vi "Measurement UI.vi"() -> ()   [LabVIEW 2021, in "audio_frequencyResponseMeasurement.lvlib"]
uses:
  audio_frequencyResponseMeasurement.lvlib
panel:
  in  "MeasGraphs":T1(tab)
  out "FrequencyResponseGraph":cluster{"X":dbl[], "Y":dbl[]}(graph) caption="AC"
  out "TimeDomainGraph":waveform(dbl)(graph) caption="AC"
  out "RMSLevelGraph":cluster{"X":dbl[], "Y":dbl[]}(graph) caption="AC"
  out "THDResponseGraph":cluster{"X":dbl[], "Y":dbl[]}(graph) caption="AC"
  out "THD+NResponseGraph":cluster{"X":dbl[], "Y":dbl[]}(graph) caption="AC"
  out "THD+N response":dbl[](array[numeric])
  out "Frequency response":dbl[](array[numeric])
  out "Time domain":dbl[](array[numeric])
  out "dt":dbl
  in  "Analog source resource name":string
  in  "Protocol capture channel":string="0L" caption="Channel list"
  out "RMS levels":dbl[](array[numeric])
  out "Harmonics levels":dbl[](array[numeric])
  out "THD response":dbl[](array[numeric])
  out "Frequency steps":dbl[](array[numeric])
  in  "Data line":u16 caption="DATA LINE"
  in  "Channel":u32 caption="CHANNEL"
  in  "MeasSettingsOptions":i32(listbox)=-1
  in  "Settling time":dbl caption="SETTLING TIME" format="%#_6ps"
  in  "Setting cycles":i32 caption="SETTLING CYCLES"
  in  "Maximum harmonic":i32=5 caption="MAX HARMONIC"
  in  "DC Offset":dbl caption="DC OFFSET" format="%#_6pV"
  out "Calculated sample rate":u32 caption="SAMPLE RATE" format="%#.6pHz"
  in  "Trigger source":T2(ring) caption="TRIGGER SOURCE"
  in  "Protocol capture resource name":string caption="RESOURCE NAME"
  out "Protocol settings":string="Protocol settings"
  in  "Clock rate":u32=2822400 caption="CLOCK RATE" format="%#.6pHz"
  in  "Frequency spacing":enum16{"Linear", "Logarithmic"}(ring)=enum."Logarithmic" caption="FREQUENCY SPACING"
  in  "Measurement duration":dbl=0.001 caption="MEASUREMENT DURATION" format="%#_6ps"
  in  "Measurement cycles":i32=10 caption="MEASUREMENT CYCLES"
  in  "Frequency steps":i32=20 caption="FREQUENCY STEPS"
  out "Analog source":string="Analog source "
  in  "DSGResourceName":tag="<Select Device>" caption="RESOURCE NAME"
  in  "Amplitude":dbl=-1.0 caption="AMPLITUDE" format="%#_6pdB"
  in  "Full scale range":dbl=3.16 caption="FULL SCALE RANGE" format="%.3pV"
  in  "Frequency stop":dbl=10000.0 caption="FREQUENCY STOP" format="%#_6pHz"
  in  "Frequency start":dbl=100.0 caption="FREQUENCY START" format="%#_6pHz"
  out "Measurement settings":string="Measurement settings"
  in  "MeasSettings":bool
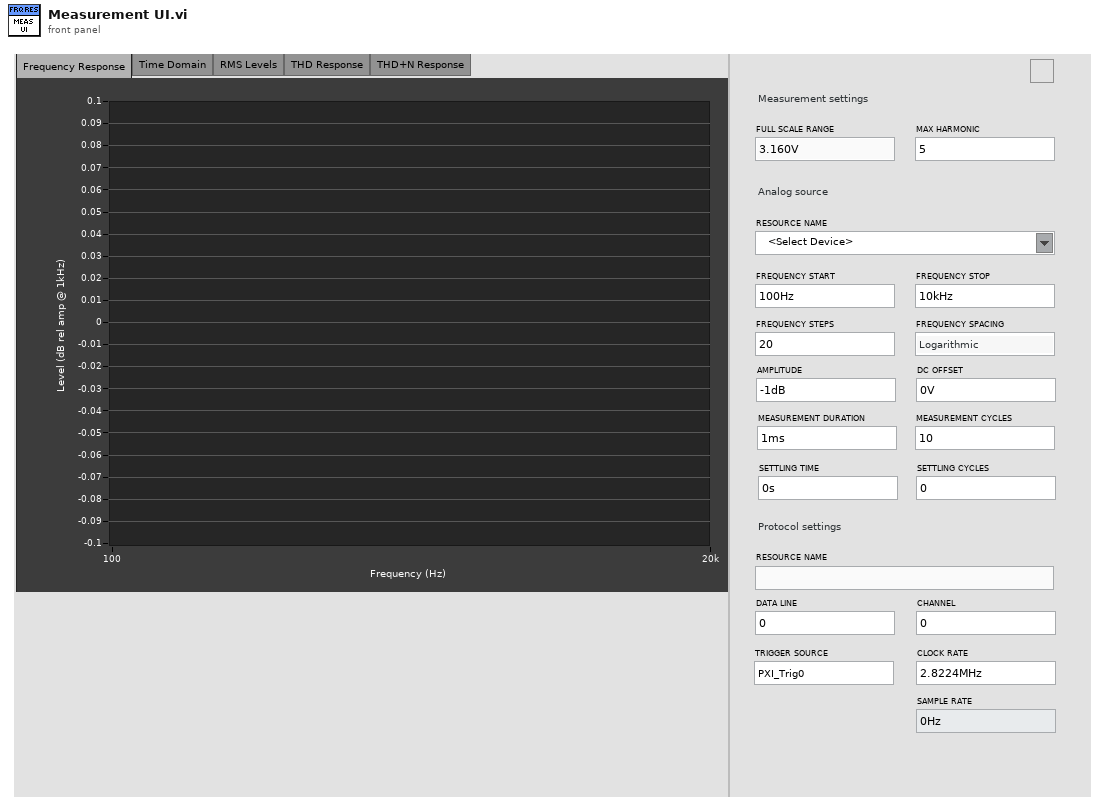
[diagram p1: front panel]
types:
  T1 = enum32{"Frequency Response", "Time Domain", "RMS Levels", "THD Response", "THD+N Response", "Hidden Controls"}
  T2 = enum16{"PXI_Trig0", "PXI_Trig1", "PXI_Trig2", "PXI_Trig3", "PXI_Trig4", "PXI_Trig5", "PXI_Trig6", "PXI_Trig7"}
  T3 = enum16{"open", "replace", "create", "open or create", "replace or create", "replace or create with confirmation"}
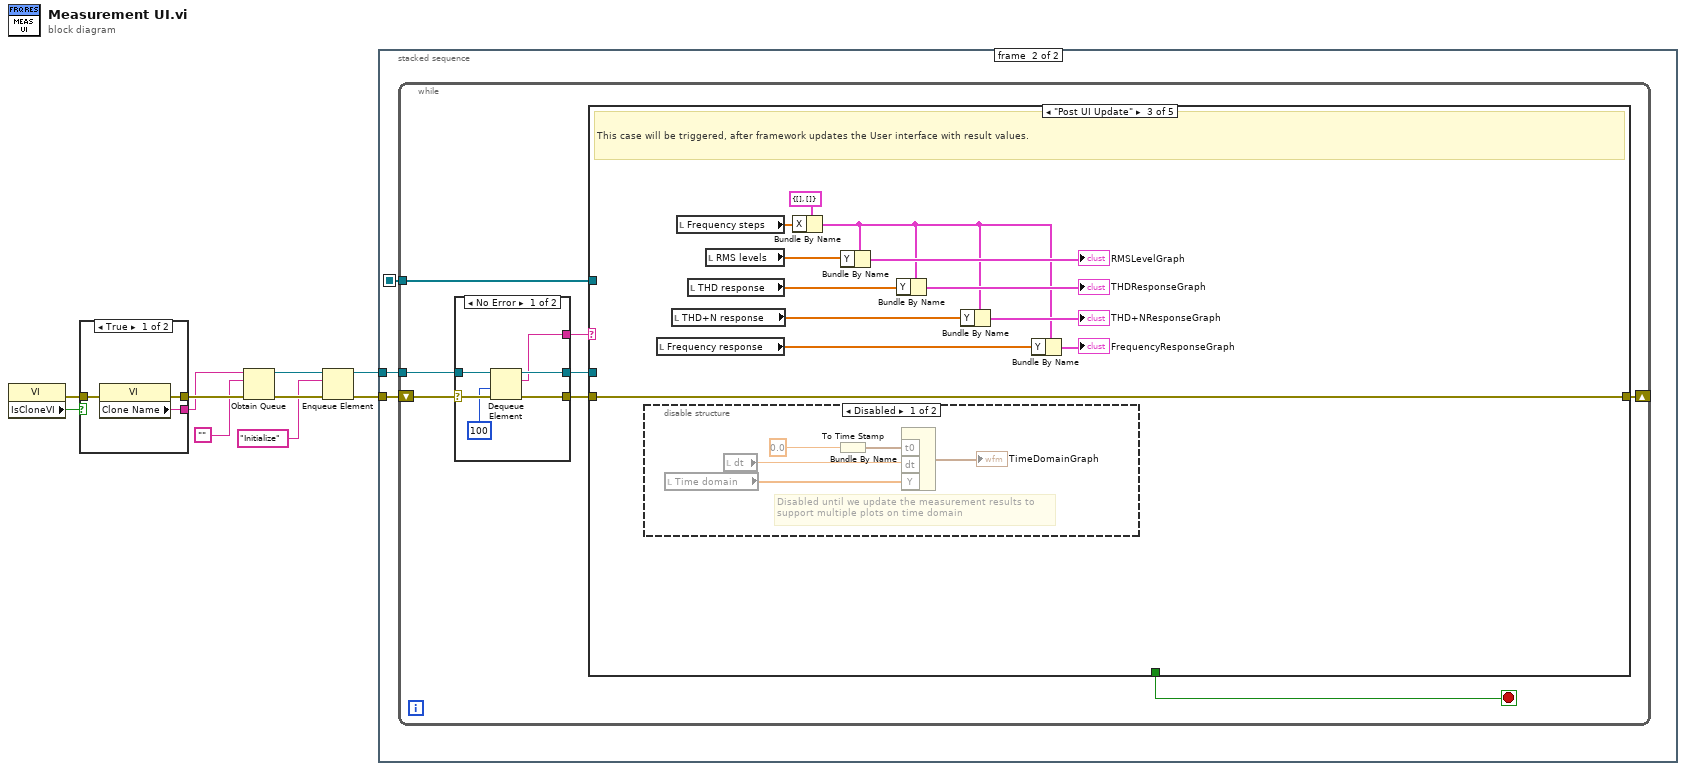
[diagram p0: block diagram]
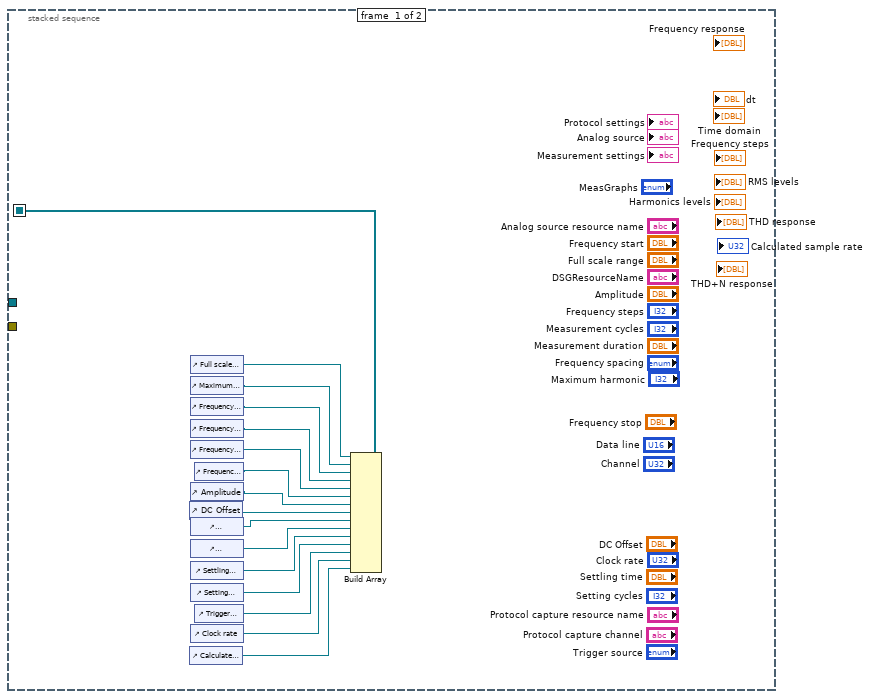
[diagram p2: hidden frame]
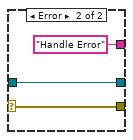
[diagram p3: hidden frame]
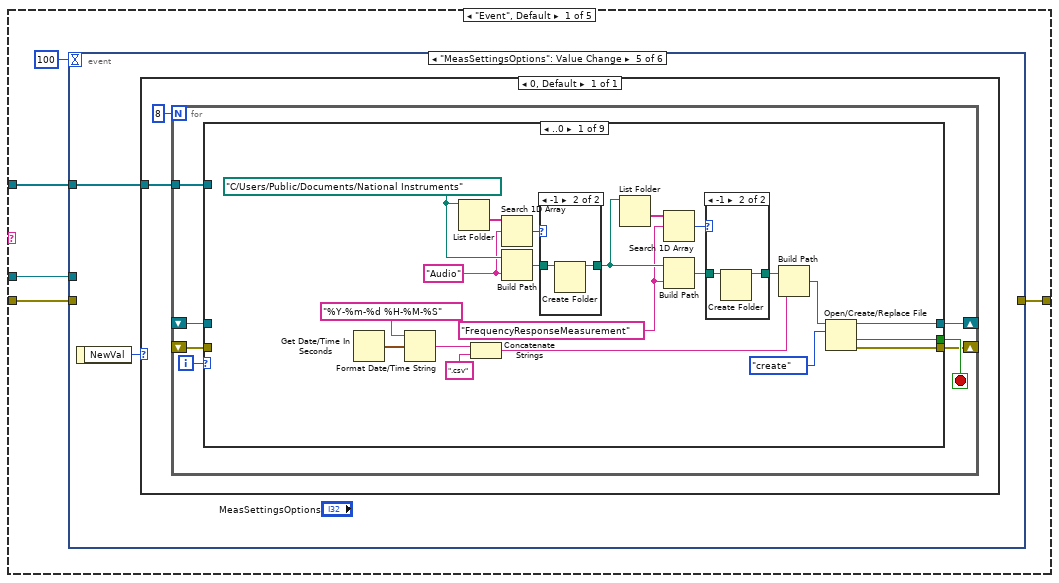
[diagram p4: hidden frame]
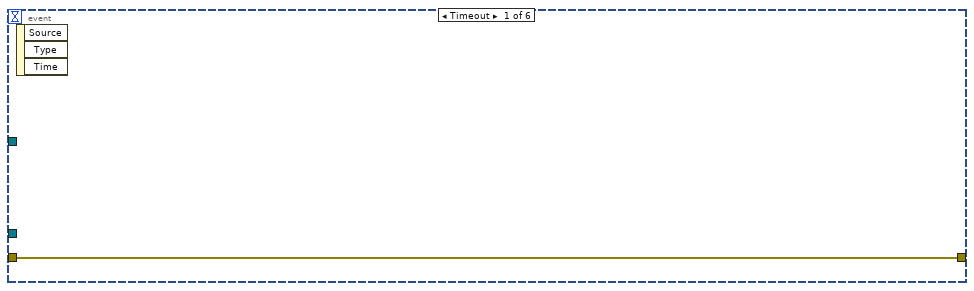
[diagram p5: hidden frame]
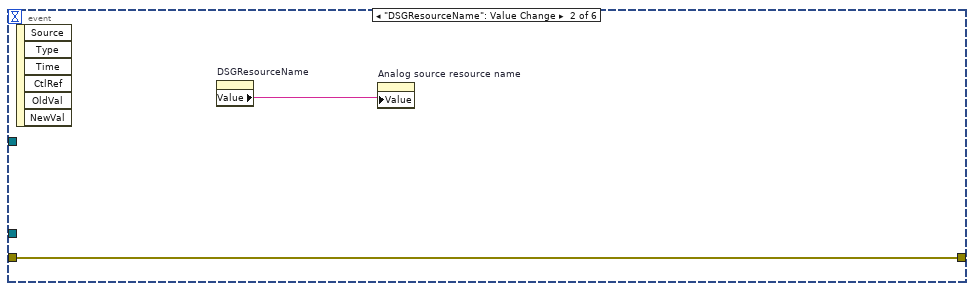
[diagram p6: hidden frame]
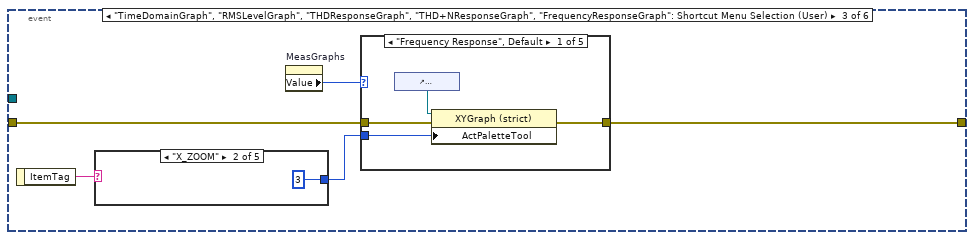
[diagram p7: hidden frame]
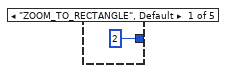
[diagram p8: hidden frame]
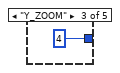
[diagram p9: hidden frame]
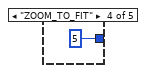
[diagram p10: hidden frame]
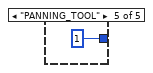
[diagram p11: hidden frame]
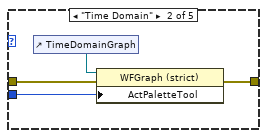
[diagram p12: hidden frame]
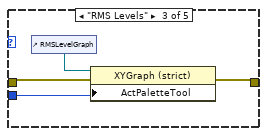
[diagram p13: hidden frame]
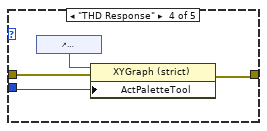
[diagram p14: hidden frame]
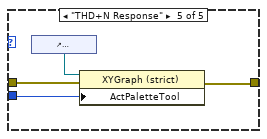
[diagram p15: hidden frame]
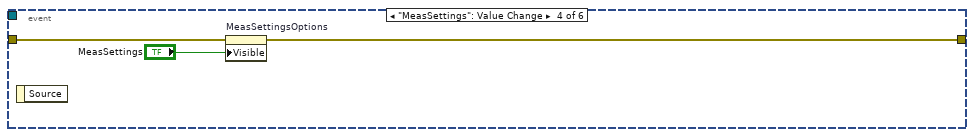
[diagram p16: hidden frame]
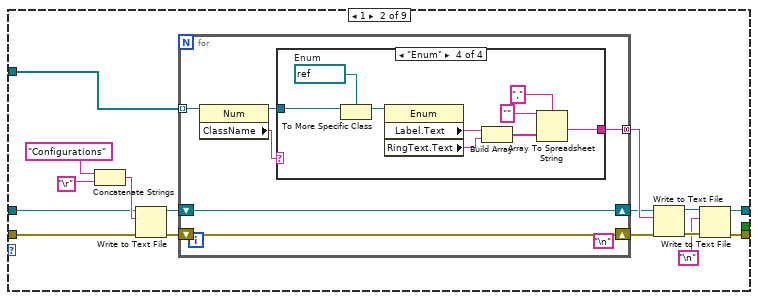
[diagram p19: hidden frame]
diagram:
  n1 = property class="VI"() -> (error out=w1:errorcluster, "IsCloneVI"=w2:bool)  [unwired: 2 in, 1 out]
  n2 = case shown="True" w2 {
    tunnel: [w13 w16] -> w10
    tunnel: [w12 w15] -> w9
    tunnel: w1 -> [w11 w14]
    frame True {
      n3 = property class="VI"(error in=w11) -> (error out=w13:errorcluster, "Clone Name"=w12:string)  [unwired: 1 in, 1 out]
    }
    frame False {
      n4 = property class="VI"(error in=w14) -> (error out=w16:errorcluster, "Name"=w15:string)  [unwired: 1 in, 1 out]
    }
  }
  n5 = Obtain Queue(name (unnamed)=w9, element data type="", error in (no error)=w10) -> (queue out=w6:refnum<queue>, error out=w8:errorcluster)  [unwired: 2 in, 1 out]
  n6 = Enqueue Element(queue=w6, element="Initialize", error in (no error)=w8) -> (queue out=w5:refnum<queue>, error out=w7:errorcluster)  [unwired: 1 in, 1 out]
  n7 = stacked-sequence {
    seq-local: [w19 _] -> [_ w33]
    tunnel: w7 -> [_ w35]
    tunnel: w5 -> [_ w34]
    frame #0 {
      n8 = control-ref of="DC Offset"() -> (w17:refnum<vi>)
      n9 = control-ref of="Calculated sample rate"() -> (w20:refnum<vi>)
      n10 = control-ref of="Full scale range"() -> (w32:refnum<vi>)
      n11 = control-ref of="Maximum harmonic"() -> (w31:refnum<vi>)
      n12 = control-ref of="Frequency start"() -> (w30:refnum<vi>)
      n13 = control-ref of="Frequency stop"() -> (w29:refnum<vi>)
      n14 = control-ref of="Frequency steps"() -> (w28:refnum<vi>)
      n15 = control-ref of="Amplitude"() -> (w18:refnum<vi>)
      n16 = control-ref of="Measurement duration"() -> (w26:refnum<vi>)
      n17 = control-ref of="Measurement cycles"() -> (w25:refnum<vi>)
      n18 = control-ref of="Settling time"() -> (w24:refnum<vi>)
      n19 = control-ref of="Setting cycles"() -> (w23:refnum<vi>)
      n20 = control-ref of="Clock rate"() -> (w21:refnum<vi>)
      n21 = control-ref of="Frequency spacing"() -> (w27:refnum<vi>)
      n22 = control-ref of="Trigger source"() -> (w22:refnum<vi>)
      n23 = Build Array(w32, w31, w30, w29, w28, w27, w18, w17, w26, w25, w24, w23, w22, w21, w20) -> (w19:refnum<vi>[])
    }
    frame #1 {
      n24 = while {
        shift-right: [w38] -> _
        shift-left: w35 -> [w43]
        tunnel: w34 -> [w41]
        tunnel: w33 -> [w36]
        stop <- w37 stop-if-true
        n25 = case shown="No Error" w43 {
          selector: w43 -> [w49 w52]
          tunnel: [w48 w52] -> w42
          tunnel: w41 -> [w47 w51]
          tunnel: [w46 w51] -> w40
          tunnel: [w45 "Handle Error"] -> w39
          frame No Error {
            n26 = Dequeue Element(queue=w47, timeout in ms (-1)=100, error in (no error)=w49) -> (queue out=w46:refnum<queue>, element=w45:string, error out=w48:errorcluster)  [unwired: 1 out]
          }
          frame Error {
          }
        }
        n27 = case shown="\"Post UI Update\"" w39 {
          tunnel: w42 -> [w56 w365 w379 w391 w392]
          tunnel: w40 -> [w54 _ _ w389 _]
          tunnel: [w57 w365 w379 w386 w392] -> w38
          tunnel: [_ _ _ TRUE _] -> w37
          tunnel: w36 -> [w53 _ _ _ _]
          frame "Event", Default {
            n28 = event shown="[4] \"MeasSettingsOptions\": Value Change" {
              selector: _ -> [_ _ _ _ _ _]
              dyn-events: _ -> [_ _ _ _ _ _]
              timeout: 100 -> [_ _ _ _ _ _]
              tunnel: [w58 w60 w61 w91 _ w354] -> w57
              tunnel: w56 -> [w58 w60 w63 w93 _ w355]
              tunnel: w54 -> [_ _ _ _ _ w353]
              tunnel: w53 -> [_ _ _ _ w95 _]
              event Timeout {
                n29 = event-data() -> ()  [unwired: 1 in, 3 out]
              }
              event "DSGResourceName": Value Change {
                n30 = event-data() -> ()  [unwired: 1 in, 6 out]
                n31 = property on="DSGResourceName" class="DAQmxName"() -> ("Value"=w59:string)  [unwired: 2 in, 2 out]
                n32 = property on="Analog source resource name" class="Str"("Value"=w59) -> ()  [unwired: 2 in, 2 out]
              }
              event "TimeDomainGraph", "RMSLevelGraph", "THDResponseGraph", "THD+NResponseGraph", "FrequencyResponseGraph": Shortcut Menu Selection (User) {
                n33 = event-data() -> ("ItemTag"=w64:string)  [unwired: 1 in]
                n34 = case shown="\"X_ZOOM\"" w64 {
                  tunnel: [2 3 4 5 1] -> w62
                  frame "ZOOM_TO_RECTANGLE", Default {
                  }
                  frame "X_ZOOM" {
                  }
                  frame "Y_ZOOM" {
                  }
                  frame "ZOOM_TO_FIT" {
                  }
                  frame "PANNING_TOOL" {
                  }
                }
                n35 = property on="MeasGraphs" class="TabCtl (strict)"() -> ("Value"=w65:T1)  [unwired: 2 in, 2 out]
                n36 = case shown="\"Frequency Response\", Default" w65 {
                  tunnel: w63 -> [w74 w77 w81 w86 w90]
                  tunnel: w62 -> [w71 w76 w80 w83 w89]
                  tunnel: [w73 w75 w79 w85 w88] -> w61
                  frame "Frequency Response", Default {
                    n37 = control-ref of="FrequencyResponseGraph"() -> (w72:refnum<vi>)
                    n38 = property class="XYGraph (strict)"(reference=w72, error in=w74, "ActPaletteTool"=w71) -> (error out=w73:errorcluster)  [unwired: 1 out]
                  }
                  frame "Time Domain" {
                    n39 = control-ref of="TimeDomainGraph"() -> (w78:refnum<vi>)
                    n40 = property class="WFGraph (strict)"(reference=w78, error in=w77, "ActPaletteTool"=w76) -> (error out=w75:errorcluster)  [unwired: 1 out]
                  }
                  frame "RMS Levels" {
                    n41 = control-ref of="RMSLevelGraph"() -> (w82:refnum<vi>)
                    n42 = property class="XYGraph (strict)"(reference=w82, error in=w81, "ActPaletteTool"=w80) -> (error out=w79:errorcluster)  [unwired: 1 out]
                  }
                  frame "THD Response" {
                    n43 = control-ref of="THDResponseGraph"() -> (w84:refnum<vi>)
                    n44 = property class="XYGraph (strict)"(reference=w84, error in=w86, "ActPaletteTool"=w83) -> (error out=w85:errorcluster)  [unwired: 1 out]
                  }
                  frame "THD+N Response" {
                    n45 = control-ref of="THD+NResponseGraph"() -> (w87:refnum<vi>)
                    n46 = property class="XYGraph (strict)"(reference=w87, error in=w90, "ActPaletteTool"=w89) -> (error out=w88:errorcluster)  [unwired: 1 out]
                  }
                }
              }
              event "MeasSettings": Value Change {
                n47 = event-data() -> ()  [unwired: 1 in, 1 out]
                n48 = property on="MeasSettingsOptions" class="LstBox (strict)"(error in=w93, "Visible"="MeasSettings") -> (error out=w91:errorcluster)  [unwired: 1 in, 1 out]
              }
              event "MeasSettingsOptions": Value Change {
                n49 = event-data() -> ("NewVal"=w94:i32)  [unwired: 1 in]
                n50 = case shown="0, Default" w94 {
                  tunnel: w95 -> [w96]
                  frame 0, Default {
                    n51 = for {
                      N: 8 -> [_]
                      shift-right: [w102] -> _
                      shift-left: _ -> [w101]
                      shift-right: [w100] -> _
                      shift-left: _ -> [w99]
                      tunnel: w96 -> [w98]
                      i -> [w104]
                      stop <- w103 stop-if-true
                      n52 = case shown="..0" w104 {
                        tunnel: [w118 _ _ _ _ _ _ _ _] -> w103
                        tunnel: [w124 w144 w188 w215 w253 w285 w317 refnum<file> refnum ("refnum out") w351] -> w102
                        tunnel: w101 -> [_ w141 w208 w226 w274 w306 w338 w349 w351]
                        tunnel: [w117 w143 w186 w214 w251 w283 w315 w347 w350] -> w100
                        tunnel: w99 -> [_ w139 w207 w227 w273 w305 w337 w346 w350]
                        tunnel: w98 -> [_ w142 _ _ _ _ _ _ _]
                        frame ..0 {
                          w113 = "FrequencyResponseMeasurement" ("prompt")
                          w120 = "Audio" ("prompt")
                          w123 = path "C:/Users/Public/Documents/National Instruments" ("base path")
                          n53 = Get Date/Time In Seconds() -> (seconds since 1Jan1904=w110:timestamp)
                          n54 = Format Date/Time String(time format string (%c)="%Y-%m-%d %H-%M-%S", seconds (now)=w110) -> (date/time string=w109:string)  [unwired: 1 in]
                          n55 = List Folder(path=w123) -> (folder names=w121:string[])  [unwired: 3 in, 3 out]
                          n56 = Concatenate Strings(w109, ".csv" ("string")) -> (w106:string)
                          n57 = Search 1D Array(1D array=w121, element=w120) -> (index of element=w119:i32)  [unwired: 1 in]
                          n58 = Build Path(base path=w123, name or relative path=w120) -> (appended path=w122:path)
                          n59 = case shown="-1" w119 {
                            tunnel: w122 -> [w129 w131]
                            tunnel: [w129 w130] -> w114
                            frame Default {
                            }
                            frame -1 {
                              n60 = Create Folder(path (use dialog)=w131) -> (created path=w130:path)  [unwired: 2 in, 2 out]
                            }
                          }
                          n61 = List Folder(path=w114) -> (folder names=w116:string[])  [unwired: 3 in, 3 out]
                          n62 = Search 1D Array(1D array=w116, element=w113) -> (index of element=w115:i32)  [unwired: 1 in]
                          n63 = Build Path(base path=w114, name or relative path=w113) -> (appended path=w112:path)
                          n64 = case shown="-1" w115 {
                            tunnel: w112 -> [w126 w128]
                            tunnel: [w126 w127] -> w107
                            frame Default {
                            }
                            frame -1 {
                              n65 = Create Folder(path (use dialog)=w128) -> (created path=w127:path)  [unwired: 2 in, 2 out]
                            }
                          }
                          n66 = Build Path(base path=w107, name or relative path=w106) -> (appended path=w105:path)
                          n67 = Open/Create/Replace File(file path (use dialog)=w105, operation (0:open)=T3."create") -> (refnum out=w124:refnum<file>, cancelled=w118:bool, error out=w117:errorcluster)  [unwired: 4 in]
                        }
                        frame 1 {
                          (unwired) "\n"
                          n68 = Concatenate Strings("Configurations" ("format string"), "\r") -> (w145:string)
                          n69 = Write to Text File(file (use dialog)=w141, text=w145, error in=w139) -> (refnum out=w138:refnum<file>, error out=w140:errorcluster)  [unwired: 1 in, 1 out]
                          n70 = for {
                            tunnel: w142 -> [w149] mode=indexing
                            shift-right: [w153] -> w136
                            shift-left: w138 -> [w153]
                            shift-right: [w152] -> w135
                            shift-left: w140 -> [w152]
                            tunnel: [w151] -> w137 mode=concatenating
                            n71 = property class="Num"(reference=w149) -> (reference out=w150:refnum<vi>, "ClassName"=w148:string)  [unwired: 1 in, 1 out]
                            n72 = case shown="\"Enum\"" w148 {
                              tunnel: [_ w157 w167 w176] -> w151
                              tunnel: w150 -> [_ w155 w165 w180]
                              frame Default {
                              }
                              frame "Digital" {
                                w154 = refnum<vi> refnum  # Digital
                                n73 = To More Specific Class(target class=w154, reference=w155) -> (specific class reference=w156:refnum<vi>)  [unwired: 1 in, 1 out]
                                n74 = property class="DigNum"(reference=w156) -> ("Label.Text"=w162:string, "NumText.Text"=w161:string)  [unwired: 1 in, 2 out]
                                n75 = Build Array(w162, w161) -> (w158:string[])
                                n76 = Array To Spreadsheet String(delimiter (Tab)=",", array=w158, 3:"" ("format string")) -> (spreadsheet string=w157:string)
                              }
                              frame "Ring" {
                                w164 = refnum<vi> refnum  # Ring
                                n77 = To More Specific Class(target class=w164, reference=w165) -> (specific class reference=w166:refnum<vi>)  [unwired: 1 in, 1 out]
                                n78 = property class="Ring"(reference=w166) -> ("Label.Text"=w163:string, "RingText.Text"=w171:string)  [unwired: 1 in, 2 out]
                                n79 = Build Array(w163, w171) -> (w168:string[])
                                n80 = Array To Spreadsheet String(delimiter (Tab)=",", array=w168, 3:"" ("format string")) -> (spreadsheet string=w167:string)
                              }
                              frame "Enum" {
                                w179 = refnum<vi> refnum  # Enum
                                n81 = To More Specific Class(target class=w179, reference=w180) -> (specific class reference=w175:refnum<vi>)  [unwired: 1 in, 1 out]
                                n82 = property class="Enum"(reference=w175) -> ("Label.Text"=w174:string, "RingText.Text"=w173:string)  [unwired: 1 in, 2 out]
                                n83 = Build Array(w174, w173) -> (w172:string[])
                                n84 = Array To Spreadsheet String(delimiter (Tab)=",", array=w172, 3:"" ("format string")) -> (spreadsheet string=w176:string)
                              }
                            }
                          }
                          n85 = Write to Text File(file (use dialog)=w136, text=w137, error in=w135) -> (refnum out=w134:refnum<file>, error out=w133:errorcluster)  [unwired: 1 in, 1 out]
                          n86 = Write to Text File(file (use dialog)=w134, text="\n", error in=w133) -> (refnum out=w144:refnum<file>, error out=w143:errorcluster)  [unwired: 1 in, 1 out]
                        }
                        frame 2 {
                          w181 = "\r"
                          n87 = property on="FrequencyResponseGraph" class="XYGraph (strict)"() -> ("Value"=w183:cluster{"X":dbl[], "Y":dbl[]})  [unwired: 2 in, 2 out]
                          n88 = Concatenate Strings("Results" ("string"), w181, "Frequency Response" ("string"), w181) -> (w205:string)
                          n89 = Write to Text File(file (use dialog)=w208, text=w205, error in=w207) -> (refnum out=w201:refnum<file>, error out=w200:errorcluster)  [unwired: 1 in, 1 out]
                          n90 = Build Array("Frequency (Hz)", "Level (dB rel amp @ 1kHz)") -> (w204:string[])
                          n91 = Unbundle By Name(w183) -> ("X"=w192:dbl[], "Y"=w193:dbl[])
                          n92 = Array To Spreadsheet String(delimiter (Tab)=",", array=w204, 3:"" ("format string")) -> (spreadsheet string=w199:string)
                          n93 = for {
                            tunnel: w192 -> [w213] mode=indexing
                            tunnel: w193 -> [w209] mode=indexing
                            tunnel: [w210] -> w194 mode=indexing
                            n94 = Format Into String(w213) -> (resulting string=w211:string)  [unwired: 3 in, 1 out]
                            n95 = Format Into String(w209) -> (resulting string=w212:string)  [unwired: 3 in, 1 out]
                            n96 = Build Array(w211, w212) -> (w210:string[])
                          }
                          n97 = Write to Text File(file (use dialog)=w201, text=w199, error in=w200) -> (refnum out=w198:refnum<file>, error out=w197:errorcluster)  [unwired: 1 in, 1 out]
                          n98 = Array To Spreadsheet String(delimiter (Tab)=",", array=w194, 3:"" ("format string")) -> (spreadsheet string=w191:string)
                          n99 = Write to Text File(file (use dialog)=w198, text=w191, error in=w197) -> (refnum out=w190:refnum<file>, error out=w189:errorcluster)  [unwired: 1 in, 1 out]
                          n100 = Write to Text File(file (use dialog)=w190, text="\n", error in=w189) -> (refnum out=w188:refnum<file>, error out=w186:errorcluster)  [unwired: 1 in, 1 out]
                        }
                        frame 3 {
                          n101 = property on="TimeDomainGraph" class="WFGraph (strict)"() -> ("Value"=w219:waveform(dbl))  [unwired: 2 in, 2 out]
                          n102 = Concatenate Strings("Time Domain" ("string"), "\r") -> (w239:string)
                          n103 = Write to Text File(file (use dialog)=w226, text=w239, error in=w227) -> (refnum out=w236:refnum<file>, error out=w235:errorcluster)  [unwired: 1 in, 1 out]
                          n104 = Build Array("Time (s)", "Amplitude (V)") -> (w238:string[])
                          n105 = Unbundle By Name(w219) -> ("dt"=w224:dbl, "Y"=w225:dbl[])
                          n106 = Array To Spreadsheet String(delimiter (Tab)=",", array=w238, 3:"" ("format string")) -> (spreadsheet string=w234:string)
                          n107 = Write to Text File(file (use dialog)=w236, text=w234, error in=w235) -> (refnum out=w233:refnum<file>, error out=w232:errorcluster)  [unwired: 1 in, 1 out]
                          n108 = for {
                            tunnel: [w245] -> w229 mode=indexing
                            tunnel: w225 -> [w244] mode=indexing
                            tunnel: w224 -> [w242]
                            i -> [w243]
                            n109 = Multiply(x=w242, y=w243) -> (x*y=w241:dbl)
                            n110 = Format Into String(w241) -> (resulting string=w246:string)  [unwired: 3 in, 1 out]
                            n111 = Format Into String(w244) -> (resulting string=w247:string)  [unwired: 3 in, 1 out]
                            n112 = Build Array(w246, w247) -> (w245:string[])
                          }
                          n113 = Array To Spreadsheet String(delimiter (Tab)=",", array=w229, 3:"" ("format string")) -> (spreadsheet string=w228:string)
                          n114 = Write to Text File(file (use dialog)=w233, text=w228, error in=w232) -> (refnum out=w217:refnum<file>, error out=w216:errorcluster)  [unwired: 1 in, 1 out]
                          n115 = Write to Text File(file (use dialog)=w217, text="\n", error in=w216) -> (refnum out=w215:refnum<file>, error out=w214:errorcluster)  [unwired: 1 in, 1 out]
                        }
                        frame 4 {
                          n116 = property on="RMSLevelGraph" class="XYGraph (strict)"() -> ("Value"=w248:cluster{"X":dbl[], "Y":dbl[]})  [unwired: 2 in, 2 out]
                          n117 = Concatenate Strings("RMS Level" ("string"), "\r") -> (w271:string)
                          n118 = Build Array("Frequency (Hz)", "Level (Vrms)") -> (w270:string[])
                          n119 = Write to Text File(file (use dialog)=w274, text=w271, error in=w273) -> (refnum out=w267:refnum<file>, error out=w266:errorcluster)  [unwired: 1 in, 1 out]
                          n120 = Array To Spreadsheet String(delimiter (Tab)=",", array=w270, 3:"" ("format string")) -> (spreadsheet string=w265:string)
                          n121 = Unbundle By Name(w248) -> ("X"=w258:dbl[], "Y"=w259:dbl[])
                          n122 = Write to Text File(file (use dialog)=w267, text=w265, error in=w266) -> (refnum out=w264:refnum<file>, error out=w263:errorcluster)  [unwired: 1 in, 1 out]
                          n123 = for {
                            tunnel: w258 -> [w279] mode=indexing
                            tunnel: w259 -> [w275] mode=indexing
                            tunnel: [w276] -> w260 mode=indexing
                            n124 = Format Into String(w279) -> (resulting string=w277:string)  [unwired: 3 in, 1 out]
                            n125 = Format Into String(w275) -> (resulting string=w278:string)  [unwired: 3 in, 1 out]
                            n126 = Build Array(w277, w278) -> (w276:string[])
                          }
                          n127 = Array To Spreadsheet String(delimiter (Tab)=",", array=w260, 3:"" ("format string")) -> (spreadsheet string=w257:string)
                          n128 = Write to Text File(file (use dialog)=w264, text=w257, error in=w263) -> (refnum out=w255:refnum<file>, error out=w254:errorcluster)  [unwired: 1 in, 1 out]
                          n129 = Write to Text File(file (use dialog)=w255, text="\n", error in=w254) -> (refnum out=w253:refnum<file>, error out=w251:errorcluster)  [unwired: 1 in, 1 out]
                        }
                        frame 5 {
                          n130 = Concatenate Strings("THD Response" ("string"), "\r") -> (w303:string)
                          n131 = property on="THDResponseGraph" class="XYGraph (strict)"() -> ("Value"=w280:cluster{"X":dbl[], "Y":dbl[]})  [unwired: 2 in, 2 out]
                          n132 = Build Array("Frequency (Hz)", "THD (dB)") -> (w302:string[])
                          n133 = Write to Text File(file (use dialog)=w306, text=w303, error in=w305) -> (refnum out=w299:refnum<file>, error out=w298:errorcluster)  [unwired: 1 in, 1 out]
                          n134 = Array To Spreadsheet String(delimiter (Tab)=",", array=w302, 3:"" ("format string")) -> (spreadsheet string=w297:string)
                          n135 = Unbundle By Name(w280) -> ("X"=w290:dbl[], "Y"=w291:dbl[])
                          n136 = Write to Text File(file (use dialog)=w299, text=w297, error in=w298) -> (refnum out=w296:refnum<file>, error out=w295:errorcluster)  [unwired: 1 in, 1 out]
                          n137 = for {
                            tunnel: w290 -> [w311] mode=indexing
                            tunnel: w291 -> [w307] mode=indexing
                            tunnel: [w308] -> w292 mode=indexing
                            n138 = Format Into String(w311) -> (resulting string=w309:string)  [unwired: 3 in, 1 out]
                            n139 = Format Into String(w307) -> (resulting string=w310:string)  [unwired: 3 in, 1 out]
                            n140 = Build Array(w309, w310) -> (w308:string[])
                          }
                          n141 = Array To Spreadsheet String(delimiter (Tab)=",", array=w292, 3:"" ("format string")) -> (spreadsheet string=w289:string)
                          n142 = Write to Text File(file (use dialog)=w296, text=w289, error in=w295) -> (refnum out=w287:refnum<file>, error out=w286:errorcluster)  [unwired: 1 in, 1 out]
                          n143 = Write to Text File(file (use dialog)=w287, text="\n", error in=w286) -> (refnum out=w285:refnum<file>, error out=w283:errorcluster)  [unwired: 1 in, 1 out]
                        }
                        frame 6 {
                          n144 = property on="THD+NResponseGraph" class="XYGraph (strict)"() -> ("Value"=w312:cluster{"X":dbl[], "Y":dbl[]})  [unwired: 2 in, 2 out]
                          n145 = Concatenate Strings("THD+N Response" ("string"), "\r") -> (w335:string)
                          n146 = Build Array("Frequency (Hz)", "THD+N (dB)") -> (w334:string[])
                          n147 = Write to Text File(file (use dialog)=w338, text=w335, error in=w337) -> (refnum out=w331:refnum<file>, error out=w330:errorcluster)  [unwired: 1 in, 1 out]
                          n148 = Array To Spreadsheet String(delimiter (Tab)=",", array=w334, 3:"" ("format string")) -> (spreadsheet string=w329:string)
                          n149 = Unbundle By Name(w312) -> ("X"=w322:dbl[], "Y"=w323:dbl[])
                          n150 = Write to Text File(file (use dialog)=w331, text=w329, error in=w330) -> (refnum out=w328:refnum<file>, error out=w327:errorcluster)  [unwired: 1 in, 1 out]
                          n151 = for {
                            tunnel: w322 -> [w343] mode=indexing
                            tunnel: w323 -> [w339] mode=indexing
                            tunnel: [w340] -> w324 mode=indexing
                            n152 = Format Into String(w343) -> (resulting string=w341:string)  [unwired: 3 in, 1 out]
                            n153 = Format Into String(w339) -> (resulting string=w342:string)  [unwired: 3 in, 1 out]
                            n154 = Build Array(w341, w342) -> (w340:string[])
                          }
                          n155 = Array To Spreadsheet String(delimiter (Tab)=",", array=w324, 3:"" ("format string")) -> (spreadsheet string=w321:string)
                          n156 = Write to Text File(file (use dialog)=w328, text=w321, error in=w327) -> (refnum out=w319:refnum<file>, error out=w318:errorcluster)  [unwired: 1 in, 1 out]
                          n157 = Write to Text File(file (use dialog)=w319, text="\n", error in=w318) -> (refnum out=w317:refnum<file>, error out=w315:errorcluster)  [unwired: 1 in, 1 out]
                        }
                        frame 7 {
                          w345 = FALSE ("Visible")
                          n158 = Close File(refnum=w349, error in=w346) -> (error out=w347:errorcluster)  [unwired: 1 out]
                          n159 = property on="MeasSettingsOptions" class="LstBox (strict)"("Visible"=w345, "Value"=-1 ("MeasSettingsOptions")) -> ()  [unwired: 2 in, 2 out]
                          n160 = property on="MeasSettings" class="Bool (strict)"("Value"=w345) -> ()  [unwired: 2 in, 2 out]
                        }
                        frame Default {
                        }
                      }
                    }
                  }
                }
              }
              event Panel Close? {
                n161 = event-data() -> ()  [unwired: 1 in, 4 out]
                n162 = Enqueue Element(queue=w353, element="Exit", error in (no error)=w355) -> (error out=w354:errorcluster)  [unwired: 1 in, 2 out]
                n163 = event-data("Discard?"=TRUE) -> ()  [unwired: 1 in, 1 out]
              }
            }
          }
          frame "Initialize" {
            n164 = control-ref of="TimeDomainGraph"() -> (w358:refnum<vi>)
            n165 = control-ref of="THD+NResponseGraph"() -> (w357:refnum<vi>)
            n166 = control-ref of="THDResponseGraph"() -> (w362:refnum<vi>)
            n167 = control-ref of="RMSLevelGraph"() -> (w361:refnum<vi>)
            n168 = control-ref of="FrequencyResponseGraph"() -> (w360:refnum<vi>)
            n169 = Build Array(w360, w362, w361, w357) -> (w363:refnum<vi>[])
            n170 = for {
              tunnel: w363 -> [w367] mode=indexing
              n171 = property class="XYGraph (strict)"(reference=w367, "ActPaletteTool"=2 ("Palette:Active Tool")) -> ()  [unwired: 1 in, 2 out]
            }
            n172 = property class="WFGraph (strict)"(reference=w358, "ActPaletteTool"=2 ("Palette:Active Tool")) -> ()  [unwired: 1 in, 2 out]
            n173 = property on="DSGResourceName" class="DAQmxName"("Value"="<Select Device>") -> ()  [unwired: 2 in, 2 out]
          }
          frame "Post UI Update" {
            # "This case will be triggered, after framework updates the User interface with result values."
            n174 = disable-structure shown="Disabled" {
              frame Disabled {
                # "Disabled until we update the measurement results to\nsupport multiple plots on time domain"
                n175 = local read "Time domain"() -> (w383:dbl[])
                n176 = local read "dt"() -> (w380:dbl)
                n177 = To Time Stamp(1:0.0 ("t0")) -> (0:w381:timestamp)
                n178 = Bundle By Name("t0"=w381, "dt"=w380, "Y"=w383) -> (→"TimeDomainGraph":waveform(dbl))  [unwired: 1 in]
              }
              frame Enabled {
              }
            }
            n179 = local read "Frequency response"() -> (w378:dbl[])
            n180 = local read "THD+N response"() -> (w371:dbl[])
            n181 = local read "Frequency steps"() -> (w376:dbl[])
            n182 = local read "THD response"() -> (w372:dbl[])
            n183 = local read "RMS levels"() -> (w369:dbl[])
            n184 = Bundle By Name(cluster=cluster{"X":dbl[], "Y":dbl[]} {"X"=[], "Y"=[]} ("THD vs Amplitude"), "X"=w376) -> (w368:cluster{"X":dbl[], "Y":dbl[]})
            n185 = Bundle By Name(cluster=w368, "Y"=w369) -> (→"RMSLevelGraph":cluster{"X":dbl[], "Y":dbl[]})
            n186 = Bundle By Name(cluster=w368, "Y"=w372) -> (→"THDResponseGraph":cluster{"X":dbl[], "Y":dbl[]})
            n187 = Bundle By Name(cluster=w368, "Y"=w371) -> (→"THD+NResponseGraph":cluster{"X":dbl[], "Y":dbl[]})
            n188 = Bundle By Name(cluster=w368, "Y"=w378) -> (→"FrequencyResponseGraph":cluster{"X":dbl[], "Y":dbl[]})
          }
          frame "Exit" {
            # "This case is triggered to close the User Interface from framework"
            n189 = Flush Queue(queue=w389, error in (no error)=w391) -> (queue out=w388:refnum<queue>, error out=w387:errorcluster)  [unwired: 1 out]
            n190 = Release Queue(queue=w388, force destroy? (F)=TRUE, error in (no error)=w387) -> (error out=w386:errorcluster)  [unwired: 2 out]
          }
          frame "Handle Error" {
          }
        }
      }
    }
  }
